vi "ProcessAnalogTachometer.vi"(8 "error in (no error)":errorcluster, 10 "waveform":waveform(sgl), 11 "tachometer":T1) -> (0 "error out":errorcluster, 1 "instanteous speed (RPM)":dbl, 2 "speed position info":T4, 3 "tachometer out":T1)   [LabVIEW 2017, in "CmsVirtualChannel.lvlib"]
uses:
  <vilib>/addons/InsightCM/Devices/Shared/Cms/CmsVirtualChannel/CmsVirtualChannel.lvlib
  <vilib>/addons/Sound and Vibration/Order Analysis/Misc/OAT Position Info.ctl
  <vilib>/addons/InsightCM/Devices/Shared/Cms/CmsVirtualChannel/controls/Tachometer.ctl
  <vilib>/addons/InsightCM/Utilities/Analysis/Vibration/controls/Tachometer.ctl
  <vilib>/addons/InsightCM/Utilities/Analysis/Vibration/controls/DigitalTachometer.ctl
  <vilib>/addons/InsightCM/Utilities/Analysis/Vibration/VibrationAnalysisFunctions.lvlib
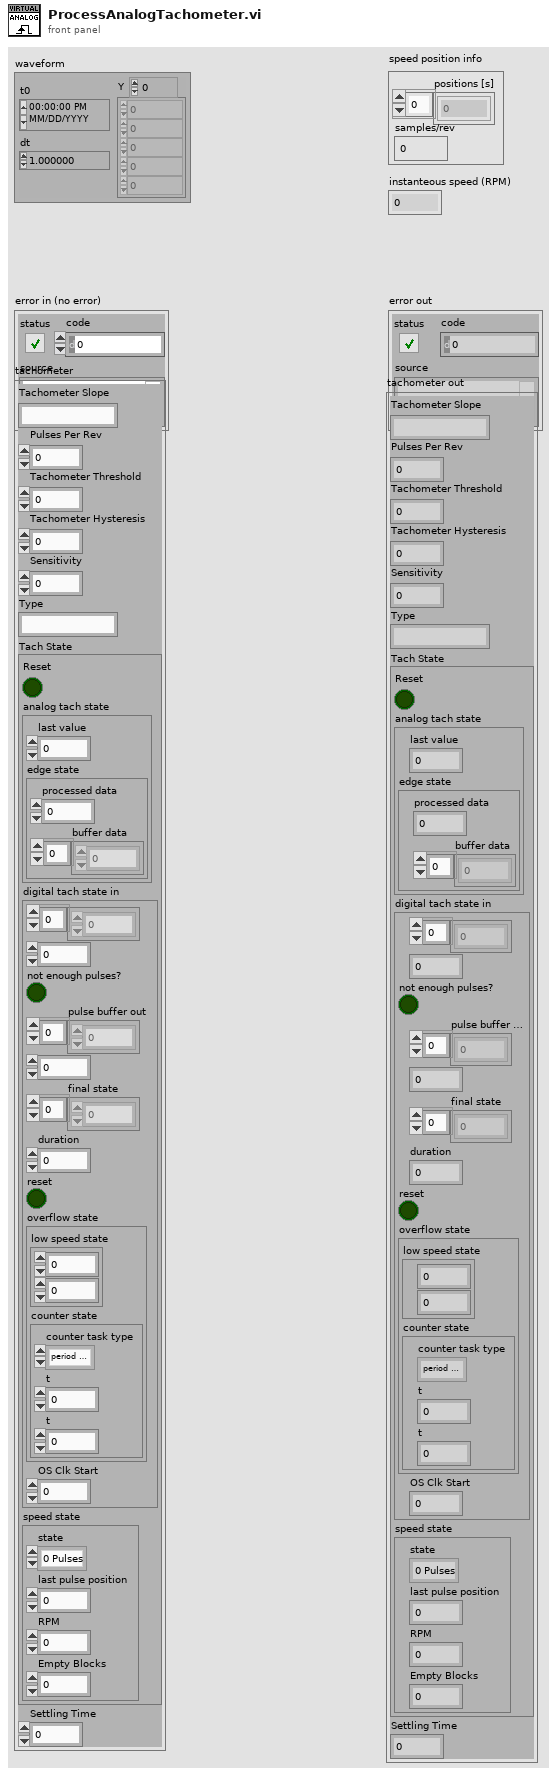
[diagram p1: front panel]
types:
  T1 = typedef "CmsVirtualChannel.lvlib/Tachometer.ctl" = cluster{"Tachometer Slope":string, "Pulses Per Rev":i32, "Tachometer Threshold":dbl, "Tachometer Hysteresis":dbl, "Sensitivity":dbl, "Type":string, "Tach State":T2, "Settling Time":dbl}
  T2 = typedef "VibrationAnalysisFunctions.lvlib/Tachometer.ctl" = cluster{"Reset":bool, "analog tach state":cluster{"last value":dbl, "edge state":cluster{"processed data":dbl, "buffer data":dbl[]}}, "digital tach state in":T3, "speed state":cluster{"state":enum16{"0 Pulses", "1 Pulse", "2+ Pulses"}, "last pulse position":dbl, "RPM":dbl, "Empty Blocks":i32}}
  T3 = typedef "VibrationAnalysisFunctions.lvlib/DigitalTachometer.ctl" = cluster{dbl[], i32, "not enough pulses?":bool, "pulse buffer out":dbl[], i32, "final state":dbl[], "duration":dbl, "reset":bool, "overflow state":cluster{"low speed state":cluster{dbl, ext}, "counter state":cluster{"counter task type":enum16{"period measurement", "event counting"}, "t":dbl, "t":dbl}}, "OS Clk Start":dbl}
  T4 = typedef "OAT Position Info.ctl" = cluster{"positions [s]":dbl[], "samples/rev":dbl}
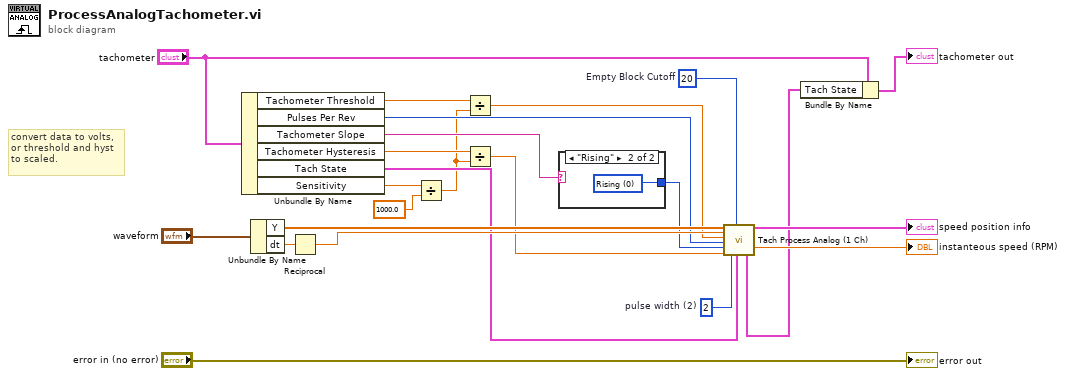
[diagram p0: block diagram]
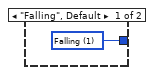
[diagram p2: hidden frame]
diagram:
  w14 = 2  # pulse width (2)
  w17 = 20  # Empty Block Cutoff
  # "convert data to volts,\nor threshold and hyst\nto scaled."
  n1 = Unbundle By Name("tachometer") -> ("Tachometer Threshold"=w3:dbl, "Pulses Per Rev"=w13:i32, "Tachometer Slope"=w12:string, "Tachometer Hysteresis"=w5:dbl, "Tach State"=w11:T2, "Sensitivity"=w7:dbl)
  n2 = Unbundle By Name("waveform") -> ("Y"=w23:sgl[], "dt"=w22:dbl)
  n3 = Reciprocal(x=w22) -> (1/x=w21:dbl)
  n4 = Divide(x=w7, y=1000.0) -> (x/y=w2:dbl)
  n5 = Divide(x=w3, y=w2) -> (x/y=w1:dbl)
  n6 = Divide(x=w5, y=w2) -> (x/y=w4:dbl)
  n7 = case shown="\"Rising\"" w12 {
    tunnel: [w24 w25] -> w18
    frame "Falling", Default {
      w24 = u16 1 items=["Rising", "Falling"] ("slope (Rising)")
    }
    frame "Rising" {
      w25 = u16 0 items=["Rising", "Falling"] ("slope (Rising)")
    }
  }
  n8 = call <vilib>:"Tach Process Analog (1 Ch).vi"("analog tacho signal"=w23, "sampling rate [Hz]"=w21, "threshold"=w1, "pulse/revolution (1)"=w13, "slope (Rising)"=w18, "hysteresis (0)"=w4, "pulse width (2)"=w14, "Empty Block Cutoff"=w17, "tach state in"=w11) -> ("tach state out"=w9:T2, "speed position info"=→"speed position info":T4, "Instant RPM"=→"instanteous speed (RPM)":dbl)  [unwired: 7 in, 1 out]
  n9 = Bundle By Name(cluster="tachometer", "Tach State"=w9) -> (→"tachometer out":T1)
  "error out" <- "error in (no error)"
